vi "MainCameraViewLoop.vi"(11 "Framerate (Hz)":i32=25) -> ()   [LabVIEW 2011]
uses:
  CIGrabControlMsg.ctl
  CIGrabControlMsgEnum.ctl
  CIGrabParams.ctl
  qtrk/QTrkLVBinding/QTrkInstance.ctl
  qtrk/QTrkLVBinding/ResultManagerInstance.ctl
  GlobalVariables.vi
panel:
  in  "Run main grab loop?":bool=TRUE
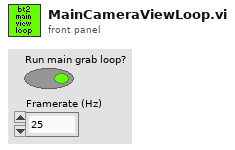
[diagram p1: front panel]
types:
  T1 = typedef "CIGrabControlMsg.ctl" = cluster{"Msg":T2}
  T2 = typedef "CIGrabControlMsgEnum.ctl" = enum16{"Stop", "EnableTracking", "DisableTracking"}
  T3 = typedef "CIGrabParams.ctl" = cluster{"QTrk Instance":T4, "ResultManager":T5, "Send to queue?":bool, "Force full-frame capture":bool}
  T4 = typedef "QTrkInstance.ctl" = cluster{"QTrk Pointer":u64}
  T5 = typedef "ResultManagerInstance.ctl" = cluster{"InstancePtr":u64}
  T6 = typedef "CameraInstance.ctl" = cluster{"VI refs":T7, "Camera state":variant}
  T7 = typedef "CameraInterface.ctl" = cluster{"Close":T8, "Get/Set generic config":T9, "Grab":T10, "Show Settings Dialog":T11, "AdjustBeadPos":T12, "Save/load camera settings":T13}
  T8 = typedef "CICloseType.ctl" = refnum<vi>
  T9 = typedef "CIGetSetGenericConfig.ctl" = refnum<vi>
  T10 = typedef "CIGrabType.ctl" = refnum<vi>
  T11 = typedef "CISettingsDlg.ctl" = refnum<vi>
  T12 = typedef "CIAdjustBeadPos.ctl" = refnum<vi>
  T13 = typedef "CISaveLoadSettings.ctl" = refnum<vi>
  T14 = typedef "MeasureConfigType.ctl" = cluster{"Bead locations":cluster{"X":i32, "Y":i32}[], "ROI":i32, "Experiment base path":path, "Image output subdir":string, "Output mode":T15, "Traces output subdir":string, "QTrk Settings":T16, "Tracking Config":T17, "Experiment Name":string, "Program":T20, "ZLUT":sgl[][][], "Camera settings":T27, "Experiment Script":string, "Max frames in memory":i32, "Save traces as binary":bool, "Pixel Calibration Gain Image":string, "Pixel Calibration Offset Image":string, "Use pixel calibration images":bool, "Internal camera settings":string, "Trace write interval":i32}
  T15 = typedef "MeasureConfigOutputMode.ctl" = enum16{"None", "Track", "SaveImages"}
  T16 = typedef "QTrkSettings.ctl" = cluster{"Image width":i32, "Image height":i32, "Number of threads (CPU based)":i32, "CUDA Device":i32, "COM Background correction factor":sgl, "ZLUT MinRadius":sgl, "ZLUT Radial sample density":sgl, "ZLUT Angular sample density":sgl, "ZLUT ROI Coverage":sgl, "QI Iterations":i32, "QI MinRadius":sgl, "QI Radial sample density":sgl, "QI Angular sample density":sgl, "QI ROI Coverage":sgl, "QI Angular Step \nIteration Factor":sgl, "XCOR Profile Length":i32, "XCOR Profile Width":i32, "XCOR Iterations":i32, "Gaussian 2D Fit Iterations":i32, "Gaussian 2D Sigma (pixels)":sgl, "Downsample":i32}
  T17 = typedef "TrackingConfigType.ctl" = cluster{"Number of steps":i32, "ZLUT stepsize (um)":sgl, "Z correction factor":sgl, "Start piezo Z (um)":sgl, "Pixel size (nm)":sgl, "2D Localization Type":T18, "Z Command (None)":T19, "Z Piezo scale":bool, "ZLUT Building\nimages per frame":i32}
  T18 = typedef "QTrkLocalizationType.ctl" = enum16{"Center-of-Mass", "1D Cross-Correlation", "Quadrant Interpolation", "Gaussian 2D MLE", "QI + ZLUTAlign", "ZLUTAlign", "QI + FourierLUT"}
  T19 = typedef "QTrkZCommandType.ctl" = enum16{"Nothing", "ComputeZ", "BuildRadialZLUT", "BuildImageZLUT", "RadialZLUT+ImageZLUT"}
  T20 = typedef "ExperimentProgramType.ctl" = cluster{"Commands":T21[], "Motor Axis accuracy conditions":T24, "Axis flags":T26}
  T21 = typedef "ExProgCommandType.ctl" = cluster{"cmd":T22, "axis":T23, "value/pos":dbl, "speed":dbl, "name":string}
  T22 = typedef "ExProgCommandEnumType.ctl" = enum16{"wait", "move", "acquire", "idle", "rmove", "when", "section", "stop"}
  T23 = typedef "MotorAxisEnum.ctl" = enum16{"no axis", "magrot", "magpos", "px", "py", "pz", "camx", "camy"}
  T24 = typedef "MotorPosType.ctl" = cluster{"Magnet Z":dbl, "Magnet rotation":dbl, "Camera":T25, "Piezo XY":T25, "Piezo Z":dbl, "Coil XY":T25}
  T25 = typedef "XYf.ctl" = cluster{"X":sgl, "Y":sgl}
  T26 = typedef "MotorPosFlagsType.ctl" = cluster{"Magnet Z":bool, "Magnet rotation":bool, "Camera":cluster{"X":bool, "Y":bool}, "Piezo XY":cluster{"X":bool, "Y":bool}, "Piezo Z":bool, "Coil XY":cluster{"X":bool, "Y":bool}}
  T27 = typedef "GenericCameraConfigType.ctl" = cluster{"Framerate (Hz)":i32, "Exposure time (us)":i32, "Image size":cluster{"Width":i32, "Height":i32}, "Number of buffers":i32}
  T28 = typedef "QueueListType.ctl" = cluster{"Motor In":refnum<queue>, "User Interface Image View":refnum<queue>, "User Interface Camera Control":refnum<queue>, "User Interface Event Notifier":refnum<notifier>, "Initialized?":bool}
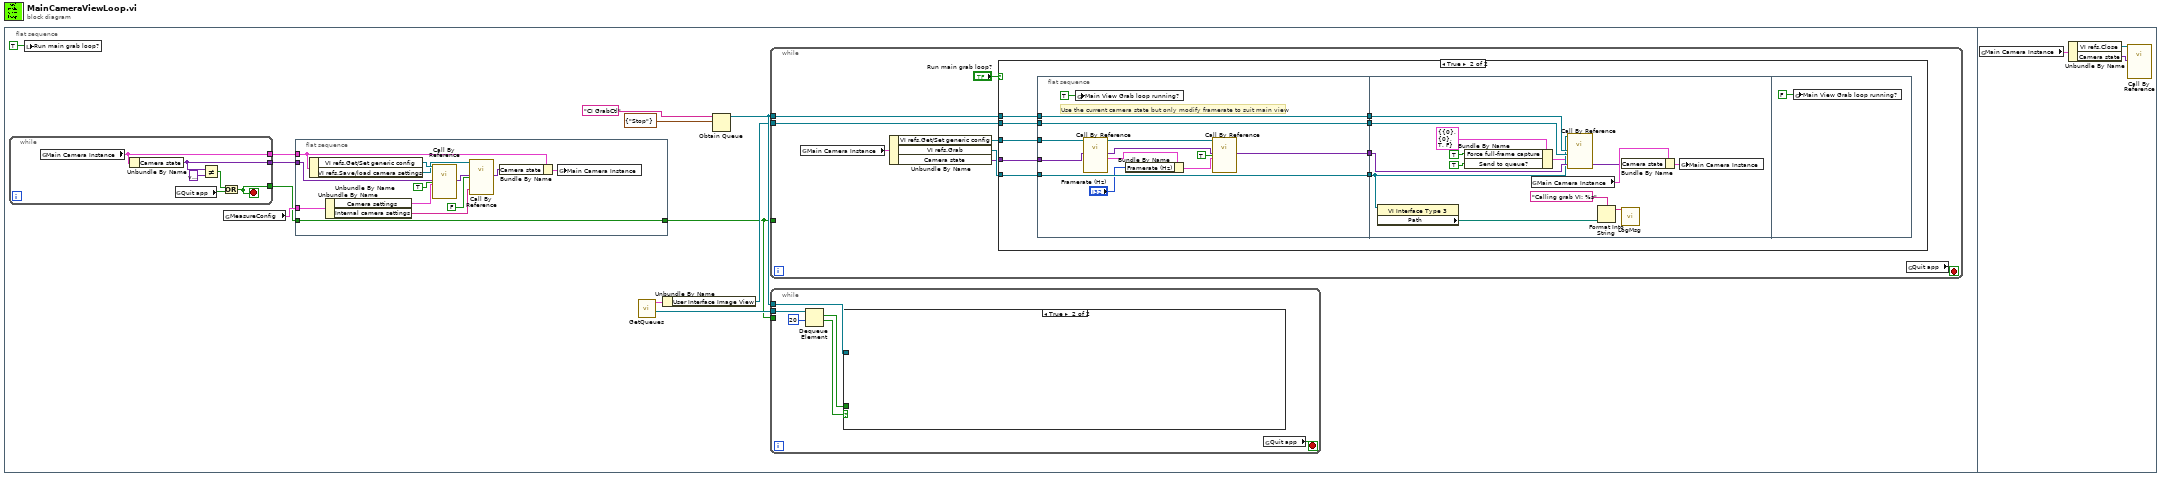
[diagram p0: block diagram]
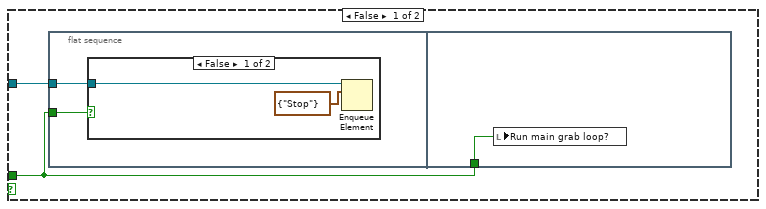
[diagram p3: hidden frame]
diagram:
  n1 = flat-sequence {
    frame #0 {
      n2 = while {
        tunnel: [w86] -> w2
        tunnel: [w85] -> w3
        tunnel: [w84] -> w4
        stop <- w86 stop-if-true
        n3 = global read "GlobalVariables.vi" "Main Camera Instance"() -> (w85:T6)
        n4 = Unbundle By Name(w85) -> ("Camera state"=w84:variant)
        n5 = global read "GlobalVariables.vi" "Quit app"() -> (w89:bool)
        n6 = Not Equal?(x=w84, y=variant ("Camera state")) -> (x != y?=w87:bool)
        n7 = Or(x=w87, y=w89) -> (x .or. y?=w86:bool)
      }
      n8 = local write "Run main grab loop?"(TRUE ("Run main grab loop?")) -> ()
      n9 = global read "GlobalVariables.vi" "MeasureConfig"() -> (w5:T14)
      n10 = flat-sequence {
        tunnel: w5 -> [w25]
        tunnel: w4 -> [w23]
        tunnel: w3 -> [w21]
        tunnel: w2 -> [w19]
        tunnel: [w19] -> w1
        frame #0 {
          n11 = Unbundle By Name(w21) -> ("VI refs.Get/Set generic config"=w24:T9, "VI refs.Save/load camera settings"=w17:T13)
          n12 = Unbundle By Name(w25) -> ("Camera settings"=w22:T27, "Internal camera settings"=w14:string)
          n13 = call-by-ref "?"(reference=w24, "Set? (F)"=TRUE, "GenericCameraConfig"=w22, "Camera state"=w23) -> ("Camera state (out)"=w16:variant)  [unwired: 8 in, 3 out]
          n14 = call-by-ref "?"(reference=w17, "Save?"=FALSE, "Serialized data"=w14, "Camera data"=w16) -> ("Camera data (out)"=w15:variant)  [unwired: 8 in, 3 out]
          n15 = Bundle By Name(cluster=w21, "Camera state"=w15) -> (w20:T6)
          n16 = global write "GlobalVariables.vi" "Main Camera Instance"(w20) -> ()
        }
      }
      n17 = call "GetQueues.vi"() -> ("User Interface Camera Control"=w7:refnum<queue>, "Queue List"=w9:T28)  [unwired: 10 in]
      n18 = Unbundle By Name(w9) -> ("User Interface Image View"=w8:refnum<queue>)
      n19 = Obtain Queue(name (unnamed)="CI GrabCtl", element data type=T1 {"Msg"=enum."Stop"} ("GrabControlMsg")) -> (queue out=w10:refnum<queue>)  [unwired: 3 in, 2 out]
      n20 = while {
        tunnel: w10 -> [w31]
        tunnel: w8 -> [w29]
        tunnel: w1 -> [_]
        stop <- w28 stop-if-true
        n21 = global read "GlobalVariables.vi" "Main Camera Instance"() -> (w27:T6)
        n22 = Unbundle By Name(w27) -> ("VI refs.Get/Set generic config"=w26:T9, "VI refs.Grab"=w32:T10, "Camera state"=w30:variant)
        n23 = case shown="True" "Run main grab loop?" {
          tunnel: w32 -> [_ w42]
          tunnel: w31 -> [_ w41]
          tunnel: w30 -> [_ w40]
          tunnel: w29 -> [_ w39]
          tunnel: w26 -> [_ w35]
          frame False {
          }
          frame True {
            n24 = flat-sequence {
              tunnel: w39 -> [w53]
              tunnel: w40 -> [w50]
              tunnel: w41 -> [w54]
              tunnel: w42 -> [w55]
              tunnel: [w55] -> w38
              tunnel: [w54] -> w37
              tunnel: [w53] -> w36
              tunnel: w35 -> [w51]
              tunnel: [w46] -> w34
              tunnel: w38 -> [w63]
              tunnel: w37 -> [w69]
              tunnel: w36 -> [w64]
              tunnel: w34 -> [w68]
              frame #0 {
                # "Use the current camera state but only modify framerate to suit main view"
                n25 = global write "GlobalVariables.vi" "Main View Grab loop running?"(TRUE ("Main View Grab loop running?")) -> ()
                n26 = call-by-ref "?"(reference=w51, "Camera state"=w50) -> (reference out=w43:T9, "GenericCameraConfig (out)"=w49:T27, "Camera state (out)"=w47:variant)  [unwired: 10 in, 1 out]
                n27 = Bundle By Name(cluster=w49, "Framerate (Hz)"="Framerate (Hz)") -> (w44:T27)
                n28 = call-by-ref "?"(reference=w43, "Set? (F)"=TRUE, "GenericCameraConfig"=w44, "Camera state"=w47) -> ("Camera state (out)"=w46:variant)  [unwired: 8 in, 3 out]
              }
              frame #1 {
                n29 = property class="VI Interface Type 3"(reference=w63) -> ("Path"=w61:path)  [unwired: 1 in, 2 out]
                n30 = Bundle By Name(cluster=T3 {"QTrk Instance"={"QTrk Pointer"=0}, "ResultManager"={"InstancePtr"=0}, "Send to queue?"=TRUE, "Force full-frame capture"=FALSE} ("TrackingParameters"), "Force full-frame capture"=TRUE, "Send to queue?"=TRUE) -> (w58:T3)
                n31 = global read "GlobalVariables.vi" "Main Camera Instance"() -> (w67:T6)
                n32 = call-by-ref "?"(reference=w63, "Camera data"=w68, "TrackingParameters"=w58, "Output Queue"=w64, "GrabControlQueue"=w69) -> ("Camera (out)"=w66:variant)  [unwired: 8 in, 2 out]
                n33 = Format Into String(format string="Calling grab VI: %s", w61) -> (resulting string=w62:string)  [unwired: 2 in, 1 out]
                n34 = Bundle By Name(cluster=w67, "Camera state"=w66) -> (w65:T6)
                n35 = call "LogMsg.vi"("msg"=w62) -> ()  [unwired: 11 in]
                n36 = global write "GlobalVariables.vi" "Main Camera Instance"(w65) -> ()
              }
              frame #2 {
                n37 = global write "GlobalVariables.vi" "Main View Grab loop running?"(FALSE ("Main View Grab loop running?")) -> ()
              }
            }
          }
        }
        n38 = global read "GlobalVariables.vi" "Quit app"() -> (w28:bool)
      }
      n39 = while {
        tunnel: w10 -> [w73]
        tunnel: w7 -> [w72]
        tunnel: w1 -> [_]
        stop <- w71 stop-if-true
        n40 = Dequeue Element(queue=w72, timeout in ms (-1)=20) -> (element=w74:bool, timed out?=w75:bool)  [unwired: 1 in, 2 out]
        n41 = case shown="True" w75 {
          tunnel: w74 -> [w77 _]
          tunnel: w73 -> [w78 _]
          frame False {
            n42 = flat-sequence {
              tunnel: w78 -> [w80]
              tunnel: w77 -> [w79]
              tunnel: w77 -> [w83]
              frame #0 {
                n43 = case shown="False" w79 {
                  tunnel: w80 -> [w82 _]
                  frame False {
                    n44 = Enqueue Element(queue=w82, element=T1 {"Msg"=enum."Stop"}) -> ()  [unwired: 2 in, 3 out]
                  }
                  frame True {
                  }
                }
              }
              frame #1 {
                n45 = local write "Run main grab loop?"(w83) -> ()
              }
            }
          }
          frame True {
          }
        }
        n46 = global read "GlobalVariables.vi" "Quit app"() -> (w71:bool)
      }
    }
    frame #1 {
      n47 = global read "GlobalVariables.vi" "Main Camera Instance"() -> (w92:T6)
      n48 = Unbundle By Name(w92) -> ("VI refs.Close"=w91:T8, "Camera state"=w90:variant)
      n49 = call-by-ref "?"(reference=w91, "Camera data"=w90) -> ()  [unwired: 12 in, 2 out]
    }
  }
